vi "Device VI 1.3.vi"() -> ()   [LabVIEW 2017]
uses:
  <vilib>/Utility/error.llb/DialogType.ctl
  <vilib>/DAQmx/read.llb/DAQmx Read (Analog 1D Wfm NChan NSamp).vi
  <vilib>/DAQmx/create/channels.llb/DAQmx Create Channel (AI-Force-Bridge-Two-Point-Linear).vi
  <vilib>/DAQmx/configure/timing.llb/DAQmx Timing (Sample Clock).vi
  <vilib>/DAQmx/configure/trigger.llb/DAQmx Start Trigger (Digital Edge).vi
  <vilib>/DAQmx/configure/trigger.llb/DAQmx Start Trigger (Analog Edge).vi
  <vilib>/DAQmx/miscellaneous.llb/DAQmx Fill In Error Info.vi
  <resource>/objmgr/daqmx.rc
panel:
  in  "Pause":bool
  in  "Start":bool
  in  "Stop 3":bool
  in  "Spreadsheet Location":path=path "C:/Users/Julio/Desktop/Device Data/Test 2.xlsx" caption="Filename"
  in  "Maximum Force":dbl=100.0
  in  "Minimum Force":dbl=-100.0
  in  "Units (Force)":i32(ring)=15875 items=["Newtons"=15875, "Pounds"=15876, "kgf"=15877, "From Custom Scale"=10065]
  in  "Trigger Type":T1(tab)
  in  "Digital Start Trigger Edge":i32(ring)=10280 caption="Edge" items=["Rising"=10280, "Falling"=10171]
  in  "Digital Start Trigger Source":tag="OnboardClock" caption="Source"
  in  "Digital Pause Trigger Pause When":i32(ring)=10192 caption="Pause When" items=["High"=10192, "Low"=10214]
  in  "Digital Pause Trigger Source":tag="/Dev1/PFI0" caption="Source"
  in  "Analog Start Trigger Level":dbl caption="Level" format="%0.2f"
  in  "Analog Start Trigger Hysteresis":dbl caption="Hysteresis" format="%.2f"
  in  "Analog Start Trigger Slope":i32(ring)=10280 caption="Slope" items=["Rising"=10280, "Falling"=10171]
  in  "Analog Start Trigger Source":string="APFI0" caption="Source"
  in  "Analog Pause Trigger Source":string="APFI0" caption="Source"
  in  "Analog Pause Trigger Pause When":i32(ring)=10093 caption="Pause When" items=["Above Level"=10093, "Below Level"=10107]
  in  "Analog Pause Trigger Level":dbl caption="Level" format="%.2f"
  in  "Bridge Information":T2={"Bridge Configuration"=10182, "Excitation Source"=10200, "Excitation Value"=2.5, "Nominal Resistance"=350.0} {"Excitation Source" items=["Internal"=10200, "External"=10167, "None"=10230]; "Bridge Configuration" items=["Full Bridge"=10182, "Half Bridge"=10187, "Quarter Bridge"=10270, "No Bridge"=10228]}
  in  "Physical Channel":tag="cDAQ2Mod1/ai0:cDAQ2Mod1/ai1"
  in  "Sample Rate":dbl=100.0
  in  "Samples per Loop":i32=100
  out "Waveform Chart":waveform(dbl)[](graph)=[{"t0"=timestamp(3612861041.642191 s since 1904-01-01), "dt"=0.01, "Y"=[0.0024447219040824282, 0.0024447219040824282, 0.0024447219040824282, 0.0024447219040824282, 0.0024447219040824282, 0.0024447219040824282, 0.0024447219040824282, 0.0024447219040824282, 0.0024447219040824282, 0.0024447219040824282, 0.0024447219040824282, 0.0024447219040824282, 0.0024447219040824282, 0.0024447219040824282, 0.0024447219040824282, 0.0024447219040824282, 0.0024447219040824282, 0.0024447219040824282, 0.0024447219040824282, 0.0024447219040824282, 0.0024447219040824282, 0.0024447219040824282, 0.0024447219040824282, 0.0024447219040824282, 0.0024447219040824282, 0.0024447219040824282, 0.0024447219040824282, 0.0024447219040824282, 0.0024447219040824282, 0.0024447219040824282, 0.0024447219040824282, 0.0024447219040824282, 0.0024447219040824282, 0.0024447219040824282, 0.0024447219040824282, 0.0024447219040824282, 0.0024447219040824282, 0.0024447219040824282, 0.0024447219040824282, 0.0024447219040824282, 0.0024447219040824282, 0.0024447219040824282, 0.0024447219040824282, 0.0024447219040824282, 0.0024447219040824282, 0.0024447219040824282, 0.0024447219040824282, 0.0024447219040824282, 0.0024447219040824282, 0.0024447219040824282, 0.0015133992739557955, 0.0015133992739557955, 0.0015133992739557955, 0.0015133992739557955, 0.0015133992739557955, 0.0015133992739557955, 0.0015133992739557955, 0.0015133992739557955, 0.0015133992739557955, 0.0015133992739557955, 0.0015133992739557955, 0.0015133992739557955, 0.0015133992739557955, 0.0015133992739557955, 0.0015133992739557955, 0.0015133992739557955, 0.0015133992739557955, 0.0015133992739557955, 0.0015133992739557955, 0.0015133992739557955, 0.0015133992739557955, 0.0015133992739557955, 0.0015133992739557955, 0.0015133992739557955, 0.0015133992739557955, 0.0015133992739557955, 0.0015133992739557955, 0.0015133992739557955, 0.0015133992739557955, 0.0015133992739557955, 0.0015133992739557955, 0.0015133992739557955, 0.0015133992739557955, 0.0015133992739557955, 0.0015133992739557955, 0.0015133992739557955, 0.0015133992739557955, 0.0015133992739557955, 0.0015133992739557955, 0.0015133992739557955, 0.0015133992739557955, 0.0015133992739557955, 0.0015133992739557955, 0.0015133992739557955, 0.0015133992739557955, 0.0015133992739557955, 0.0015133992739557955, 0.0015133992739557955, 0.0015133992739557955, 0.0015133992739557955], "attributes"=variant("NI_ChannelName"=variant(string "cDAQ2Mod1/ai0"), "NI_UnitDescription"=variant(string "Pounds"))}, {"t0"=timestamp(3612861041.642191 s since 1904-01-01), "dt"=0.01, "Y"=[0.002654269495860919, 0.002654269495860919, 0.002654269495860919, 0.002654269495860919, 0.002654269495860919, 0.002654269495860919, 0.002654269495860919, 0.002654269495860919, 0.002654269495860919, 0.002654269495860919, 0.002654269495860919, 0.002654269495860919, 0.002654269495860919, 0.002654269495860919, 0.002654269495860919, 0.002654269495860919, 0.002654269495860919, 0.002654269495860919, 0.002654269495860919, 0.002654269495860919, 0.002654269495860919, 0.002654269495860919, 0.002654269495860919, 0.002654269495860919, 0.002654269495860919, 0.002654269495860919, 0.002654269495860919, 0.002654269495860919, 0.002654269495860919, 0.002654269495860919, 0.002654269495860919, 0.002654269495860919, 0.002654269495860919, 0.002654269495860919, 0.002654269495860919, 0.002654269495860919, 0.002654269495860919, 0.002654269495860919, 0.002654269495860919, 0.002654269495860919, 0.002654269495860919, 0.002654269495860919, 0.002654269495860919, 0.002654269495860919, 0.002654269495860919, 0.002654269495860919, 0.002654269495860919, 0.002654269495860919, 0.002654269495860919, 0.002654269495860919, -0.0003725290520506384, -0.0003725290520506384, -0.0003725290520506384, -0.0003725290520506384, -0.0003725290520506384, -0.0003725290520506384, -0.0003725290520506384, -0.0003725290520506384, -0.0003725290520506384, -0.0003725290520506384, -0.0003725290520506384, -0.0003725290520506384, -0.0003725290520506384, -0.0003725290520506384, -0.0003725290520506384, -0.0003725290520506384, -0.0003725290520506384, -0.0003725290520506384, -0.0003725290520506384, -0.0003725290520506384, -0.0003725290520506384, -0.0003725290520506384, -0.0003725290520506384, -0.0003725290520506384, -0.0003725290520506384, -0.0003725290520506384, -0.0003725290520506384, -0.0003725290520506384, -0.0003725290520506384, -0.0003725290520506384, -0.0003725290520506384, -0.0003725290520506384, -0.0003725290520506384, -0.0003725290520506384, -0.0003725290520506384, -0.0003725290520506384, -0.0003725290520506384, -0.0003725290520506384, -0.0003725290520506384, -0.0003725290520506384, -0.0003725290520506384, -0.0003725290520506384, -0.0003725290520506384, -0.0003725290520506384, -0.0003725290520506384, -0.0003725290520506384, -0.0003725290520506384, -0.0003725290520506384, -0.0003725290520506384, -0.0003725290520506384], "attributes"=variant("NI_ChannelName"=variant(string "cDAQ2Mod1/ai1"), "NI_UnitDescription"=variant(string "Pounds"))}]
  # "Data"
  # "Settings"
  # "This trigger type is not supported in continuous sample timing. \n\nRefer to your device documentation for more information on which triggers are supported."
  # "This trigger type is not supported in continuous sample timing. \n\nRefer to your device documentation for more information on which triggers are supported."
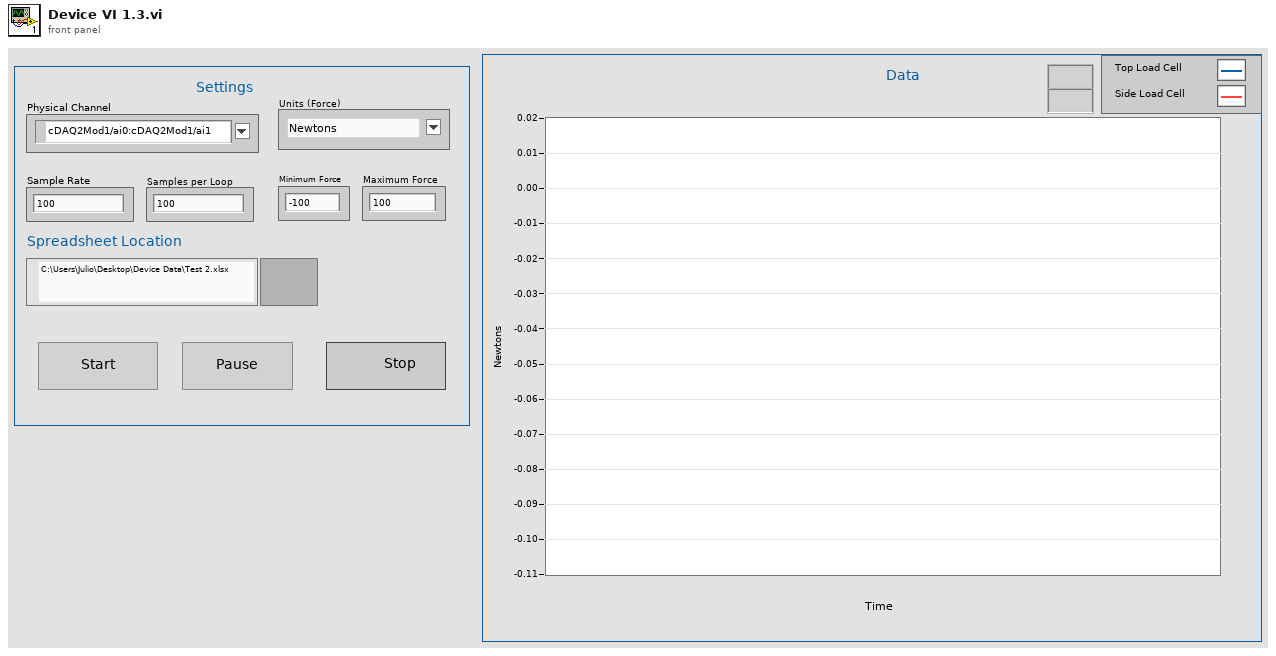
[diagram p1: front panel]
types:
  T1 = enum32{"No Trigger", "Digital Start", "Digital Pause", "Digital Reference", "Analog Start", "Analog Pause", "Analog Reference"}
  T2 = cluster{"Bridge Configuration":i32, "Excitation Source":i32, "Excitation Value":dbl, "Nominal Resistance":dbl}
  T3 = typedef "DialogType.ctl" = u16
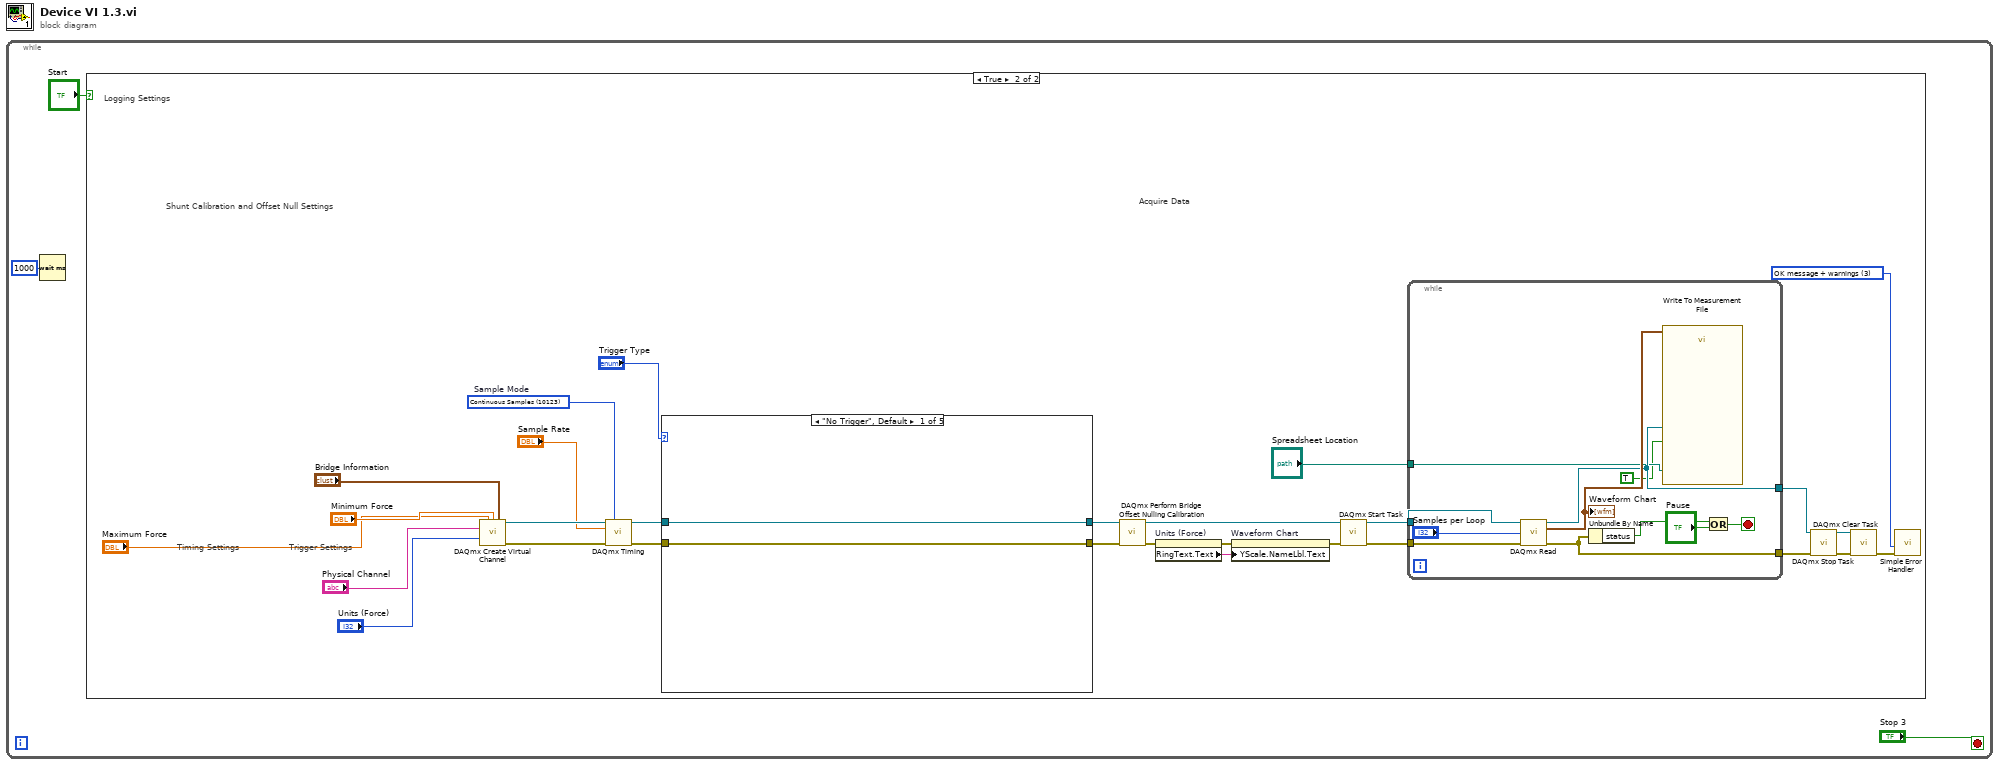
[diagram p0: block diagram]
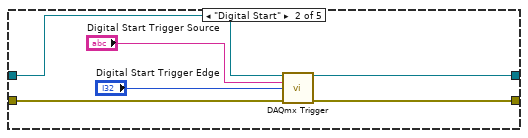
[diagram p3: hidden frame]
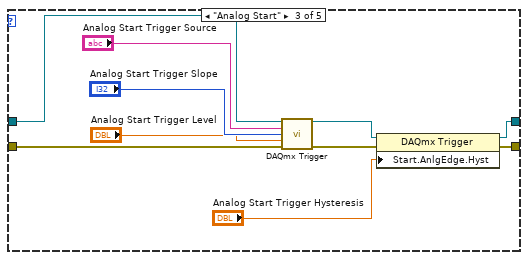
[diagram p4: hidden frame]
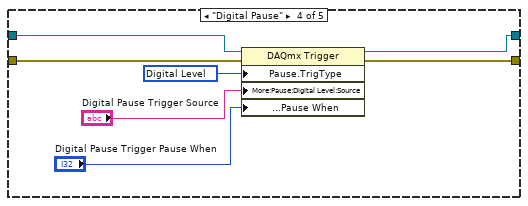
[diagram p5: hidden frame]
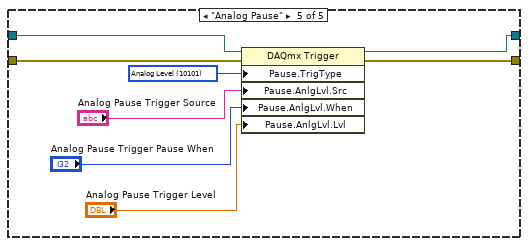
[diagram p6: hidden frame]
diagram:
  n1 = while {
    stop <- "Stop 3" stop-if-true
    n2 = Wait (ms)(milliseconds to wait=u32 1000) -> ()  [unwired: 1 out]
    n3 = case shown="True" "Start" {
      frame False {
      }
      frame True {
        w17 = T3 3 items=["no dialog", "OK message", "continue or stop message", "OK message + warnings", "continue/stop + warnings"] ("type of dialog (OK msg:1)")
        w31 = 10123 items=["Finite Samples"=10178, "Continuous Samples"=10123, "Hardware Timed Single Point"=12522]  # Sample Mode
        # "Trigger Settings"
        # "Logging Settings"
        # "Acquire Data"
        # "Shunt Calibration and Offset Null Settings"
        # "Timing Settings"
        n4 = call-poly <vilib>:"DAQmx Create Virtual Channel.vi"("maximum value"="Maximum Force", "minimum value"="Minimum Force", "bridge information"="Bridge Information", "physical channels"="Physical Channel", "units"="Units (Force)") -> ("task out"=w29:refnum<k21>, "error out"=w30:errorcluster)  [unwired: 9 in]
        n5 = call-poly <vilib>:"DAQmx Timing.vi"("task/channels in"=w29, "sample mode"=w31, "rate"="Sample Rate", "error in"=w30) -> ("task out"=w10:refnum<k21>, "error out"=w9:errorcluster)  [unwired: 10 in]
        n6 = case shown="\"No Trigger\", Default" "Trigger Type" {
          tunnel: w10 -> [w33 w39 w49 w56 w64]
          tunnel: w9 -> [w32 w38 w48 w53 w61]
          tunnel: [w33 w37 w46 w55 w63] -> w14
          tunnel: [w32 w36 w45 w54 w62] -> w15
          frame "No Trigger", Default {
          }
          frame "Digital Start" {
            n7 = call-poly <vilib>:"DAQmx Trigger.vi"("task/channels in"=w39, "source"="Digital Start Trigger Source", "edge"="Digital Start Trigger Edge", "error in"=w38) -> ("task out"=w37:refnum<k21>, "error out"=w36:errorcluster)  [unwired: 10 in]
          }
          frame "Analog Start" {
            n8 = call-poly <vilib>:"DAQmx Trigger.vi"("task/channels in"=w49, "source"="Analog Start Trigger Source", "slope"="Analog Start Trigger Slope", "level"="Analog Start Trigger Level", "error in"=w48) -> ("task out"=w44:refnum<k21>, "error out"=w43:errorcluster)  [unwired: 9 in]
            n9 = property class="DAQmx Trigger"(reference=w44, error in=w43, "Start.AnlgEdge.Hyst"="Analog Start Trigger Hysteresis") -> (reference out=w46:refnum<k21>, error out=w45:errorcluster)
          }
          frame "Digital Pause" {
            w52 = 10152 items=["Analog Level"=10101, "Analog Window"=10103, "Digital Level"=10152, "Digital Pattern"=10398, "None"=10230] ("Pause.TrigType")
            n10 = property class="DAQmx Trigger"(reference=w56, error in=w53, "Pause.TrigType"=w52, "More:Pause:Digital Level:Source"="Digital Pause Trigger Source", "More:Pause:Digital Level:Pause When"="Digital Pause Trigger Pause When") -> (reference out=w55:refnum<k21>, error out=w54:errorcluster)
          }
          frame "Analog Pause" {
            w60 = 10101 items=["Analog Level"=10101, "Analog Window"=10103, "Digital Level"=10152, "Digital Pattern"=10398, "None"=10230] ("Pause.TrigType")
            n11 = property class="DAQmx Trigger"(reference=w64, error in=w61, "Pause.TrigType"=w60, "Pause.AnlgLvl.Src"="Analog Pause Trigger Source", "Pause.AnlgLvl.When"="Analog Pause Trigger Pause When", "Pause.AnlgLvl.Lvl"="Analog Pause Trigger Level") -> (reference out=w63:refnum<k21>, error out=w62:errorcluster)
          }
        }
        n12 = call <vilib>:"DAQmx Perform Bridge Offset Nulling Calibration.vi"("task/channels in"=w14, "error in"=w15) -> ("task out"=w6:refnum<k21>, "error out"=w5:errorcluster)  [unwired: 12 in]
        n13 = property on="Units (Force)" class="Ring (strict)"(error in=w5) -> (error out=w8:errorcluster, "RingText.Text"=w7:string)  [unwired: 1 in, 1 out]
        n14 = property on="Waveform Chart" class="WFChart (strict)"(error in=w8, "YScale.NameLbl.Text"=w7) -> (error out=w23:errorcluster)  [unwired: 1 in, 1 out]
        n15 = call <vilib>:"DAQmx Start Task.vi"("task/channels in"=w6, "error in"=w23) -> ("task out"=w28:refnum<k21>, "error out"=w27:errorcluster)  [unwired: 12 in]
        n16 = while {
          tunnel: w28 -> [w75]
          tunnel: w27 -> [w74]
          tunnel: [w72] -> w20
          tunnel: [w68] -> w21
          tunnel: "Spreadsheet Location" -> [w67]
          stop <- w73 stop-if-true
          n17 = call-poly <vilib>:"DAQmx Read.vi"("task/channels in"=w75, "number of samples per channel"="Samples per Loop", "error in"=w74) -> ("task out"=w68:refnum<k21>, "data"=w69:waveform(dbl)[], "error out"=w72:errorcluster)  [unwired: 10 in]
          "Waveform Chart" <- w69
          n18 = Unbundle By Name(w72) -> ("status"=w71:bool)
          n19 = call "Write To Measurement File"("Signals"=w69, "Enable"=TRUE ("Append"), "Filename"=w67, "DAQmx Task"=w68) -> ()  [unwired: 13 in, 3 out]
          n20 = Or(x=w71, y="Pause") -> (x .or. y?=w73:bool)
        }
        n21 = call <vilib>:"DAQmx Stop Task.vi"("task/channels in"=w21, "error in"=w20) -> ("task out"=w19:refnum<k21>, "error out"=w18:errorcluster)  [unwired: 12 in]
        n22 = call <vilib>:"DAQmx Clear Task.vi"("task in"=w19, "error in"=w18) -> ("error out"=w26:errorcluster)  [unwired: 13 in]
        n23 = call <vilib>:"Simple Error Handler.vi"("type of dialog (OK msg:1)"=w17, "error in (no error)"=w26) -> ()  [unwired: 3 in, 5 out]
      }
    }
  }
